vi "custom_command.vi"() -> ()   [LabVIEW 2020]
uses:
  <vilib>/MakerHub/LINX/Public/Utilities/Open Serial.vi
  <vilib>/MakerHub/LINX/LMH-LINX.lvlib
panel:
  in  "Data":u8[](array[slide]) scale=0.0..100.0
  in  "stop":bool
  out "Response":u8[](array[slide]) scale=0.0..100.0
  in  "Serial Port":refnum<visa-resource-name>="N/A"
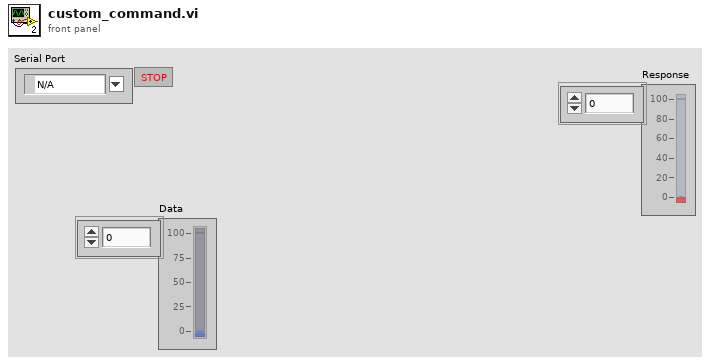
[diagram p1: front panel]
types:
  T1 = typedef "LMH-LINX.lvlib/LINX Ref.ctl" = cluster{"IO":T2, "Interface":T3, "LINX Device Config":T4}
  T2 = typedef "LMH-LINX.lvlib/Platform.ctl" = enum16{"Remote", "Local"}
  T3 = typedef "LMH-LINX.lvlib/Interface.ctl" = enum16{"Serial", "TCP"}
  T4 = typedef "LMH-LINX.lvlib/Device.lvlib/LINX Device Config.ctl" = cluster{"Interface":T3, "COM Port":refnum<visa-resource-name>, "TCP Configuration":T5, "Device Family":u8, "Device ID":u8, "Device Name":string, "TCP Ref":refnum<k5>, "Channels":T6}
  T5 = typedef "LMH-LINX.lvlib/Device.lvlib/TCP Config.ctl" = cluster{"IP Address":string, "Port":u16}
  T6 = typedef "LMH-LINX.lvlib/Channels.ctl" = cluster{"DI":u8[], "DO":u8[], "AI":u8[], "AO":u8[], "PWM":u8[], "QE":u8[], "UART":u8[], "I2C 2":u8[], "SPI":u8[], "CAN":u8[], "Servo":u8[], "AI Ref (V)":dbl, "AI Resolution (Bits)":u8, "AO Ref (V)":dbl, "AO Resolution (Bits)":u8}
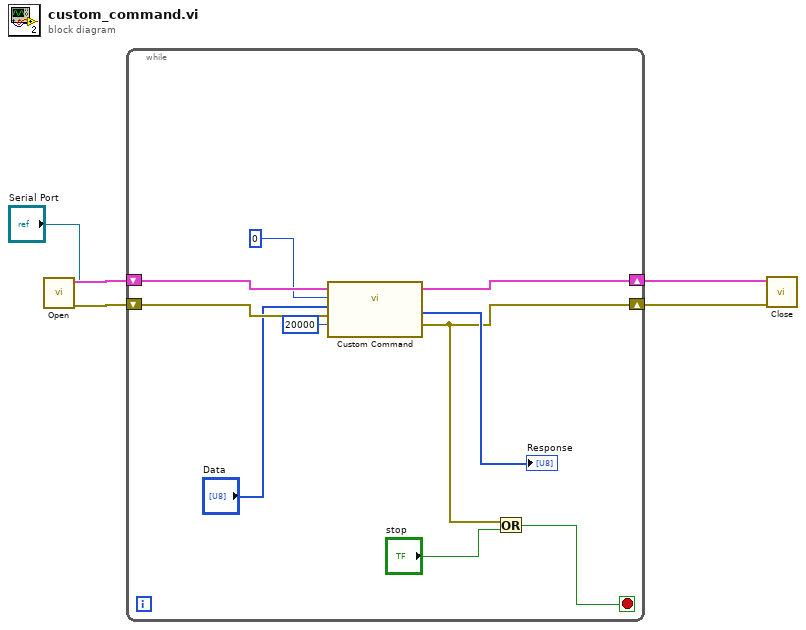
[diagram p0: block diagram]
diagram:
  n1 = call-poly <vilib>:"Open.vi"("Serial Port"="Serial Port") -> ("Error Out"=w4:errorcluster, "LINX Resource"=w5:T1)  [unwired: 8 in, 1 out]
  n2 = while {
    shift-right: [w13] -> w3
    shift-left: w5 -> [w15]
    shift-right: [w9] -> w2
    shift-left: w4 -> [w14]
    stop <- w8 stop-if-true
    n3 = call <vilib>:"Custom Command.vi"("Timeout (100 ms)"=20000, "Error In"=w14, "Data"="Data", "Custom Command Number"=u16 0, "LINX Resource"=w15) -> ("Error Out"=w9:errorcluster, "Response"=→"Response":u8[], "LINX Resource"=w13:T1)  [unwired: 3 in, 1 out]
    n4 = Or(x=w9, y="stop") -> (x .or. y?=w8:bool)
  }
  n5 = call <vilib>:"Close.vi"("Error In"=w2, "LINX Resource"=w3) -> ()  [unwired: 9 in, 1 out]
